vi "MeasureLockIn.vi"(2 "TemperatureError":dbl=200.0 format="%.2f", 3 "Temperature":dbl=200.0 format="%.2f", 4 "#Measurements each Frequency":i32=200, 5 "Path":path, 6 "error in":errorcluster, 8 "Stop":dbl=200.0 format="%.2f", 9 "Wait (ms)":dbl=200.0 format="%.2f", 10 "Step":dbl=200.0 format="%.2f", 11 "Start":dbl=200.0 format="%.2f") -> (0 "error out":errorcluster)   [LabVIEW 2010]
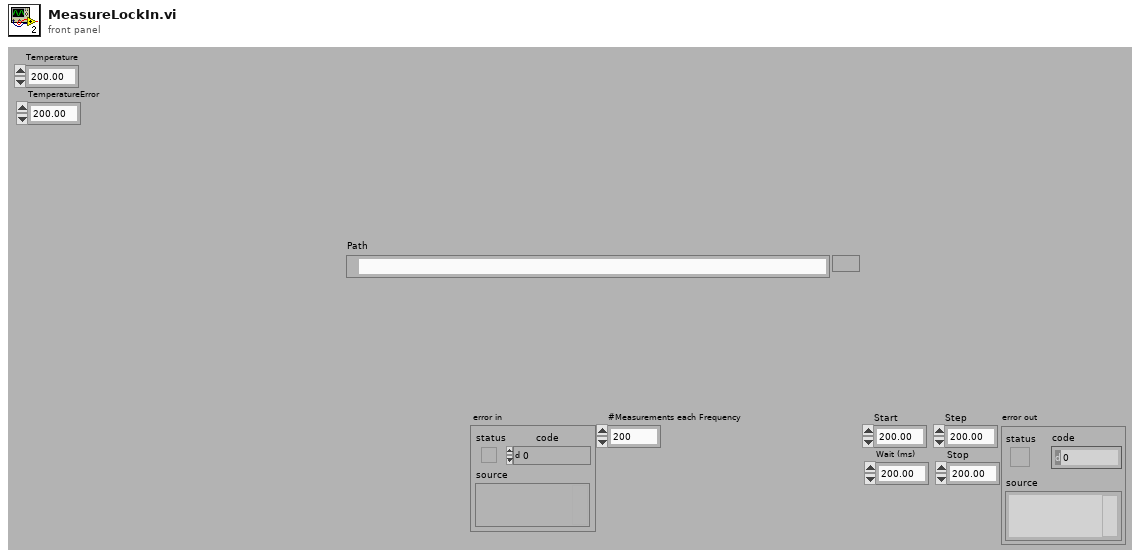
[diagram p1: front panel]
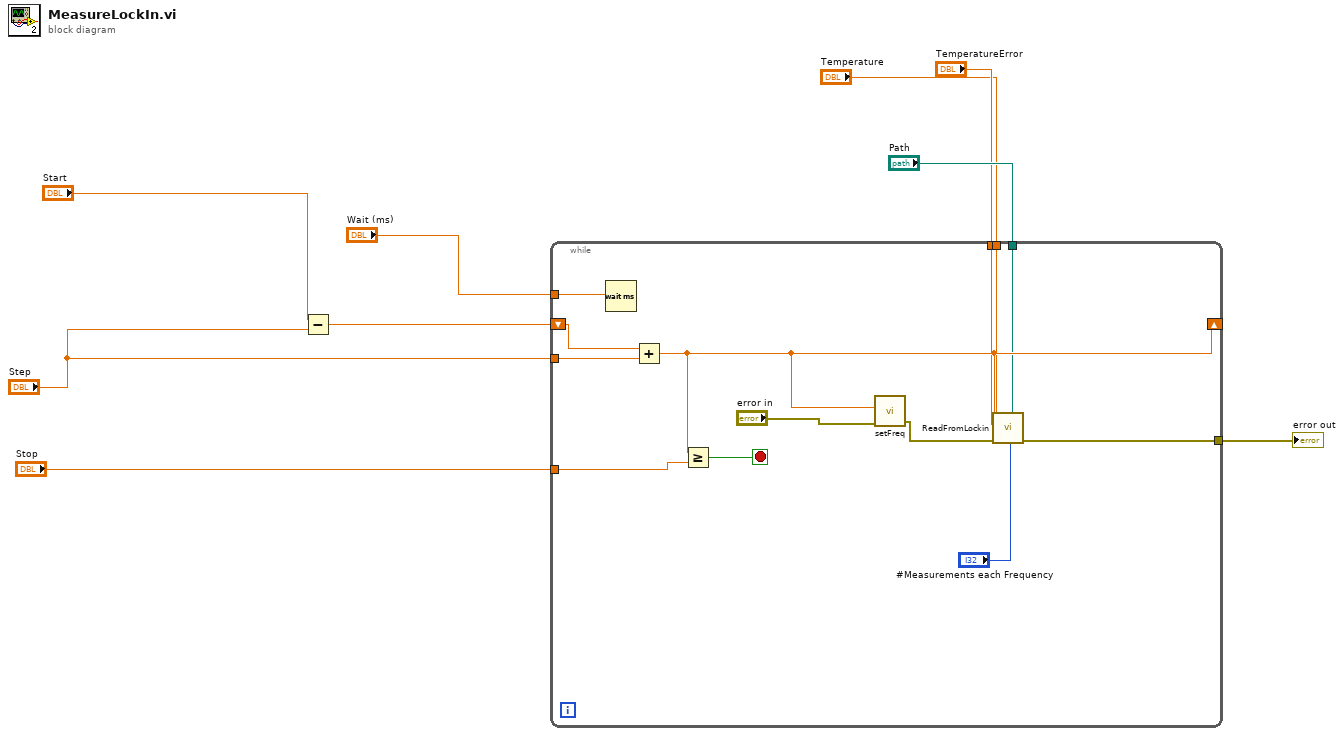
[diagram p0: block diagram]
diagram:
  n1 = Subtract(x="Start", y="Step") -> (x-y=w7:dbl)
  n2 = while {
    tunnel: "Wait (ms)" -> [w18]
    shift-right: [w16] -> _
    shift-left: w7 -> [w22]
    tunnel: "Step" -> [w21]
    tunnel: "Stop" -> [w20]
    tunnel: [w14] -> w4
    tunnel: "Path" -> [w12]
    tunnel: "TemperatureError" -> [w11]
    tunnel: "Temperature" -> [w10]
    stop <- w19 stop-if-true
    n3 = Wait (ms)(milliseconds to wait=w18) -> ()  [unwired: 1 out]
    n4 = Add(x=w22, y=w21) -> (x+y=w16:dbl)
    n5 = Greater Or Equal?(x=w16, y=w20) -> (x >= y?=w19:bool)
    n6 = call "setFreq.vi"("error in"="error in", "Frequenz in Hz"=w16) -> ("error out"=w13:errorcluster)  [unwired: 4 in]
    n7 = call "ReadFromLockin.vi"("#Measurements each Frequency"="#Measurements each Frequency", "Path"=w12, "Frequency"=w16, "error in 2"=w13, "TemperatureError"=w11, "Temperature"=w10) -> ("error out 2"=w14:errorcluster)  [unwired: 5 in]
  }
  "error out" <- w4
